vi "AM_BJT_Single_Meas.vi"(0 "VISA resource name":refnum<visa-resource-name>, 1 "Inputs":T1={"Vb / V"=0.0, "Vc / V"=0.0, "Rb / kOhm"=0.0, "Rc / kOhm"=0.0, "Delay (ms)"=500, "Nreads"=3} {"Nreads" min=3 max=50 step=1; "Delay (ms)" min=4000 max=20000 step=1}, 2 "error in (no error)":errorcluster) -> (3 "VISA resource name 2":refnum<visa-resource-name>, 4 "Raw Data":dbl[](array[numeric]), 5 "Formatted Data":dbl[](array[numeric]), 6 "error out":errorcluster)   [LabVIEW 2019]
doc: "Perform DC voltage measurement for a BJT characterisation using Arduino Micro\n\nAssumes circuit connected to Ch. A and Ch. B with BJT current amplifiers\n\nVin sourced from Ch. A, Vb sourced from Ch. B (Vb constant while Vin is swept)\n\nUse of current amplifiers means there is a voltage drop between what is set at Ch. A / Ch. B and what is sourced at Vrc-hi and Vrb-hi\n\nMeasurement (Raw Data):\nA0 = Vrc-hi, A1 = Vrc-lo, A2 = Vrb-hi, A3 = Vrb-lo, A4 = A1 = Vce, A5 = Gnd\n\nOutput (Formatted Data):\nVbin = A2, Vcin = A0, Irb = A2 - A3 / Rb, Irc = A0 - A1 / Rc, Vce = A4 - A5\n\nR. Sheehan 2 - 12 - 2020e"
panel:
  # "Measurement (Raw Data):\nA0 = Vrc-hi, A1 = Vrc-lo, A2 = Vrb-hi, A3 = Vrb-lo, A4 = A1 = Vce, A5 = Gnd\n\nOutput (Formatted Data):\nVbin = A2, Vcin = A0, Irb = A2 - A3 / Rb, Irc = A0 - A1 / Rc, Vce = A4 - A5"
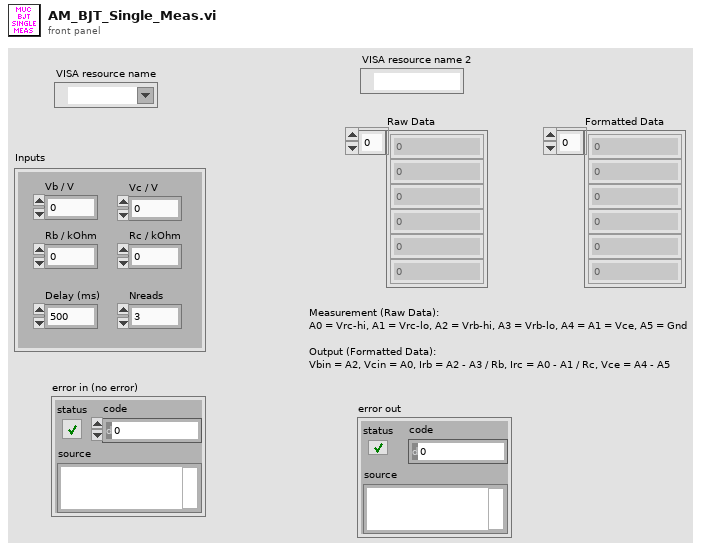
[diagram p1: front panel]
types:
  T1 = cluster{"Vb / V":dbl, "Vc / V":dbl, "Rb / kOhm":dbl, "Rc / kOhm":dbl, "Delay (ms)":u32, "Nreads":i32}
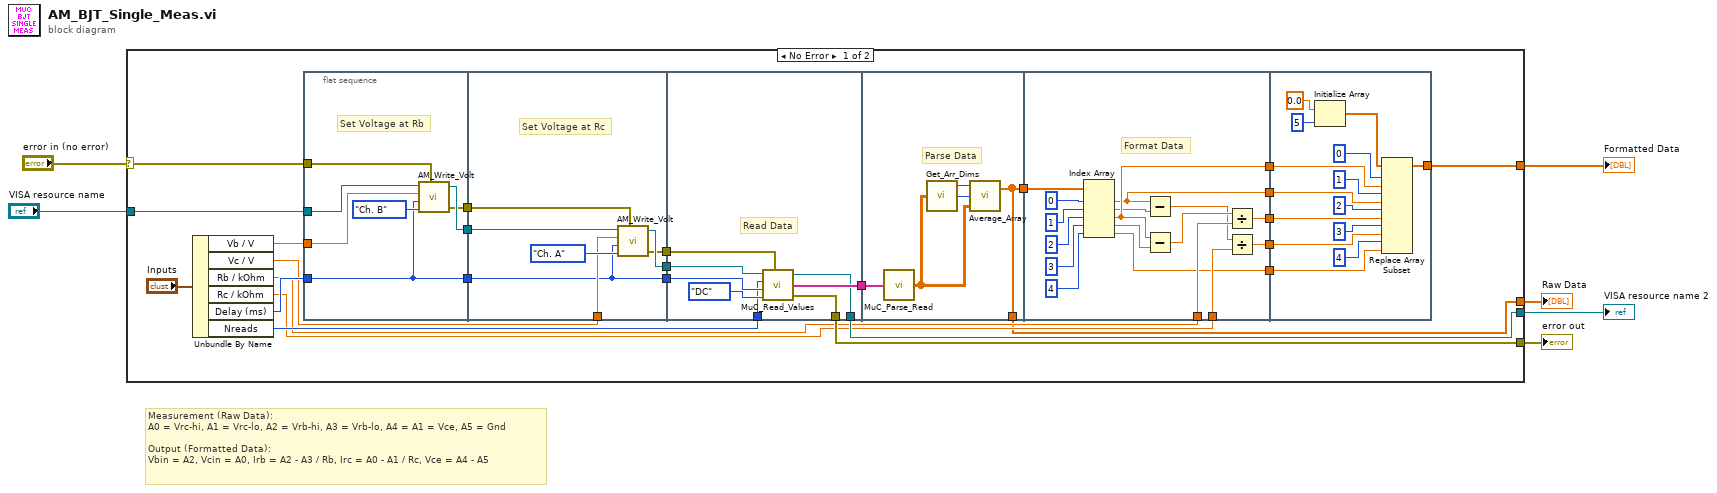
[diagram p0: block diagram]
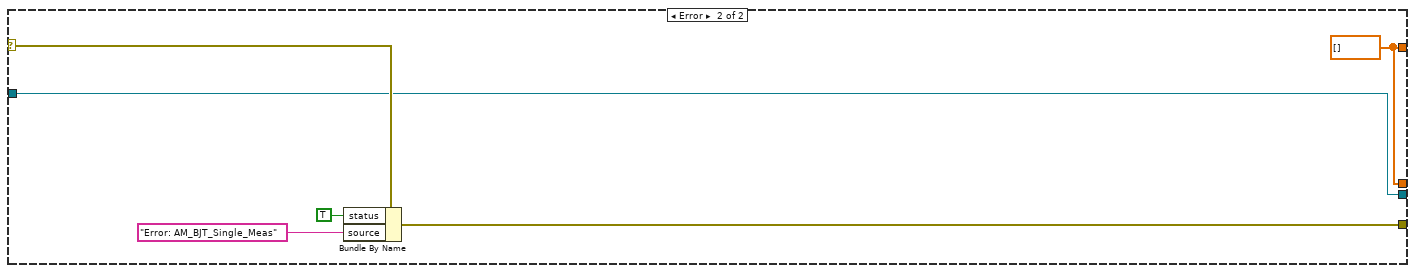
[diagram p2: hidden frame]
diagram:
  # "Measurement (Raw Data):\nA0 = Vrc-hi, A1 = Vrc-lo, A2 = Vrb-hi, A3 = Vrb-lo, A4 = A1 = Vce, A5 = Gnd\n\nOutput (Formatted Data):\nVbin = A2, Vcin = A0, Irb = A2 - A3 / Rb, Irc = A0 - A1 / Rc, Vce = A4 - A5"
  n1 = case shown="No Error" "error in (no error)" {
    selector: "error in (no error)" -> [w26 w96]
    tunnel: "VISA resource name" -> [w29 w94]
    tunnel: [w28 w94] -> w5
    tunnel: [w27 w95] -> w4
    tunnel: [w8 w91] -> w2
    tunnel: [w7 w91] -> w1
    frame No Error {
      n2 = Unbundle By Name("Inputs") -> ("Vb / V"=w22:dbl, "Vc / V"=w20:dbl, "Rb / kOhm"=w13:dbl, "Rc / kOhm"=w11:dbl, "Delay (ms)"=w21:u32, "Nreads"=w17:i32)
      n3 = flat-sequence {
        tunnel: w26 -> [w35]
        tunnel: w29 -> [w36]
        tunnel: [w38] -> w25
        tunnel: [w37] -> w24
        tunnel: w22 -> [w34]
        tunnel: w21 -> [w33]
        tunnel: [w33] -> w19
        tunnel: [w45] -> w32
        tunnel: [w44] -> w31
        tunnel: w25 -> [w43]
        tunnel: w24 -> [w42]
        tunnel: w20 -> [w41]
        tunnel: w19 -> [w40]
        tunnel: [w40] -> w18
        tunnel: w32 -> [w54]
        tunnel: w31 -> [w53]
        tunnel: [w51] -> w30
        tunnel: [w50] -> w28
        tunnel: [w49] -> w27
        tunnel: w18 -> [w48]
        tunnel: w17 -> [w47]
        tunnel: w30 -> [w56]
        tunnel: [w55] -> w16
        tunnel: [w55] -> w7
        tunnel: w16 -> [w76]
        tunnel: [w70] -> w15
        tunnel: [w65] -> w14
        tunnel: w13 -> [w67]
        tunnel: [w66] -> w12
        tunnel: w11 -> [w62]
        tunnel: [w61] -> w10
        tunnel: [w60] -> w9
        tunnel: w15 -> [w82]
        tunnel: w14 -> [w81]
        tunnel: w12 -> [w80]
        tunnel: w10 -> [w79]
        tunnel: w9 -> [w78]
        tunnel: [w77] -> w8
        frame #0 {
          # "Set Voltage at Rb"
          n4 = call "AM_Write_Volt.vi"("VISA resource name"=w36, "Volt / V"=w34, "Delay / ms"=w33, "Enum"=enum16{"Ch. A", "Ch. B"}."Ch. B", "error in (no error)"=w35) -> ("VISA resource name 2"=w38:refnum<visa-resource-name>, "error out"=w37:errorcluster)  [unwired: 1 out]
        }
        frame #1 {
          # "Set Voltage at Rc"
          n5 = call "AM_Write_Volt.vi"("VISA resource name"=w43, "Volt / V"=w41, "Delay / ms"=w40, "Enum"=enum16{"Ch. A", "Ch. B"}."Ch. A", "error in (no error)"=w42) -> ("VISA resource name 2"=w45:refnum<visa-resource-name>, "error out"=w44:errorcluster)  [unwired: 1 out]
        }
        frame #2 {
          # "Read Data"
          n6 = call "MuC_Read_Values.vi"("VISA resource name"=w54, "Nreads"=w47, "Delay (ms)"=w48, "Read Type"=enum16{"DC", "AC"}."DC", "error in (no error)"=w53) -> ("VISA resource name 2"=w50:refnum<visa-resource-name>, "Buffer Data"=w51:string[], "error out"=w49:errorcluster)
        }
        frame #3 {
          # "Parse Data"
          n7 = call "MuC_Parse_Read.vi"("Buffer Data"=w56) -> ("Data"=w59:dbl[][])
          n8 = call "Get_Arr_Dims.vi"("Data"=w59) -> ("N Rows"=w58:i32, "N Cols"=w57:i32)  [unwired: 1 out]
          n9 = call "Average_Array.vi"("Array"=w59, "Ncolumns"=w57, "Nrows"=w58) -> ("Average"=w55:dbl[])  [unwired: 1 out]
        }
        frame #4 {
          # "Format Data"
          n10 = Index Array(array=w76, index #1=0 ("index"), index #2=1 ("index"), index #3=2 ("index"), index #4=3 ("index"), index #5=4 ("index")) -> (element #1=w65:dbl, element #2=w64:dbl, element #3=w70:dbl, element #4=w69:dbl, element #5=w60:dbl)
          n11 = Subtract(x=w65, y=w64) -> (x-y=w63:dbl)
          n12 = Subtract(x=w70, y=w69) -> (x-y=w68:dbl)
          n13 = Divide(x=w68, y=w67) -> (x/y=w66:dbl)
          n14 = Divide(x=w63, y=w62) -> (x/y=w61:dbl)
        }
        frame #5 {
          n15 = Initialize Array(0.0 ("element"), 5 ("dimension size")) -> (w88:dbl[])
          n16 = Replace Array Subset(array=w88, new element #1=w82, index #1=0 ("index"), new element #2=w81, index #2=1 ("index"), new element #3=w80, index #3=2 ("index"), new element #4=w79, index #4=3 ("index"), new element #5=w78, index #5=4 ("index")) -> (w77:dbl[])
        }
      }
    }
    frame Error {
      w91 = dbl[] []
      n17 = Bundle By Name(cluster=w96, "status"=TRUE, "source"="Error: AM_BJT_Single_Meas") -> (w95:errorcluster)
    }
  }
  "VISA resource name 2" <- w5
  "error out" <- w4
  "Formatted Data" <- w2
  "Raw Data" <- w1
